vi "Create Message Accessors.vi"(7 "Message parameters":T1[](array[typedef]), 8 "error in (no error)":errorcluster, 11 "Server class in":refnum<vi>) -> (0 "error out":errorcluster, 3 "Server class out":refnum<vi>)   [LabVIEW 2019, in "gRPC Scripting Tools.lvlib"]
uses:
  gRPC Scripting Tools.lvlib
  TypeDefs/Message Metadata (Scripting).ctl
  TypeDefs/Message Element Metadata (Scripting).ctl
  TypeDefs/Message Element Type.ctl
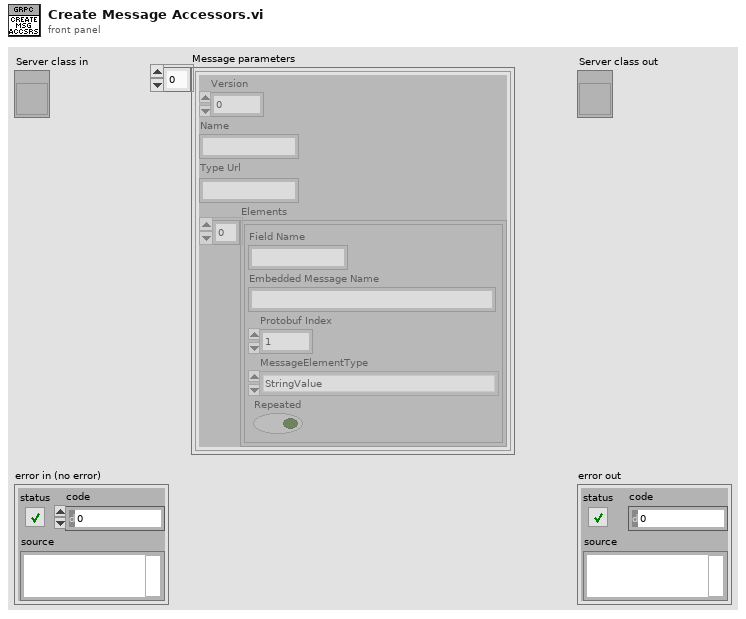
[diagram p1: front panel]
types:
  T1 = typedef "gRPC Scripting Tools.lvlib/Message Metadata (Scripting).ctl" = cluster{"Version":i32, "Name":string, "Type Url":string, "Elements":T2[]}
  T2 = typedef "gRPC Scripting Tools.lvlib/Message Element Metadata (Scripting).ctl" = cluster{"Field Name":string, "Embedded Message Name":string, "Protobuf Index":i32, "MessageElementType":T3, "Repeated":bool}
  T3 = typedef "gRPC Scripting Tools.lvlib/Message Element Type.ctl" = enum32{"Int32Value", "FloatValue", "DoubleValue", "BoolValue", "StringValue", "MessageValue", "Int64Value", "UInt32Value", "UInt64Value", "EnumValue", "Bytes", "Fixed64", "Fixed32", "SFixed64", "SFixed32", "SInt64", "SInt32"}
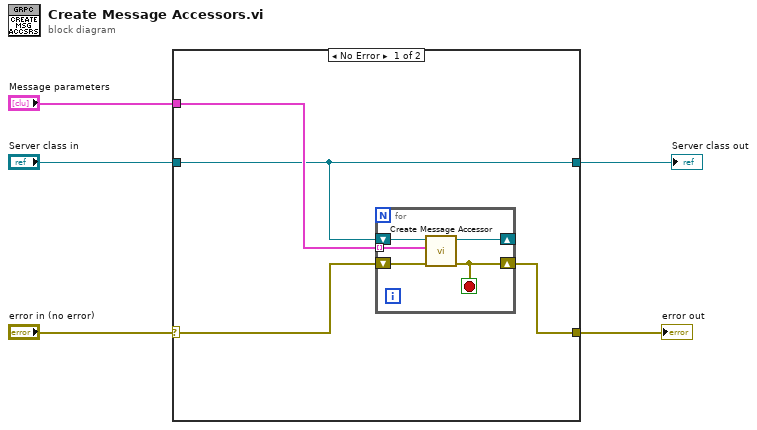
[diagram p0: block diagram]
diagram:
  n1 = case shown="No Error" "error in (no error)" {
    selector: "error in (no error)" -> [w8 w15]
    tunnel: [w7 w16] -> w5
    tunnel: "Server class in" -> [w7 w16]
    tunnel: [w6 w15] -> w3
    tunnel: "Message parameters" -> [w9 _]
    frame No Error {
      n2 = for {
        shift-right: [w11] -> w6
        shift-left: w8 -> [w14]
        shift-right: [w12] -> _
        shift-left: w7 -> [w13]
        tunnel: w9 -> [w10] mode=indexing
        stop <- w11 stop-if-true
        n3 = call "Create Message Accessor.vi"("error in (no error)"=w14, "Message Metadata"=w10, "Server class in"=w13) -> ("error out"=w11:errorcluster, "Server class out"=w12:refnum<vi>)  [unwired: 7 in]
      }
    }
    frame Error {
    }
  }
  "Server class out" <- w5
  "error out" <- w3
